vi "Write To FPGA.vi"(7 "Sample Rate":dbl, 8 "error in (no error)":errorcluster, 9 "Changed?":bool[](array[boolean]), 10 "Values":dbl[](array[numeric]), 11 "FPGA Refs":T1 {"Data Type" format="%.0x"}) -> (0 "error out":errorcluster, 2 "Values out":dbl[](array[numeric]), 3 "FPGA Refs":T1 {"Data Type" format="%.0x"})   [LabVIEW 2015, in "Fuel Injection Addon Engine.lvlib"]
uses:
  Fuel Injection Addon Engine.lvlib
  Types/FPGA Refs.ctl
  Shared/Types/FPGA Data Types.ctl
  <vilib>/rvi/errors/niLvFpgaAdjustHostInterfaceError.vi
  <vilib>/Utility/error.llb/Error Cluster From Error Code.vi
  <vilib>/rvi/interface/nirviReadWriteControl/nirviReadWriteControl.xnode
  <vilib>/rvi/interface/Simulation/niFpgaSimulationCallBeginRW.vi
  NiFpgaLv.dll
  Shared/Fuel Injection Addon Shared.lvlib
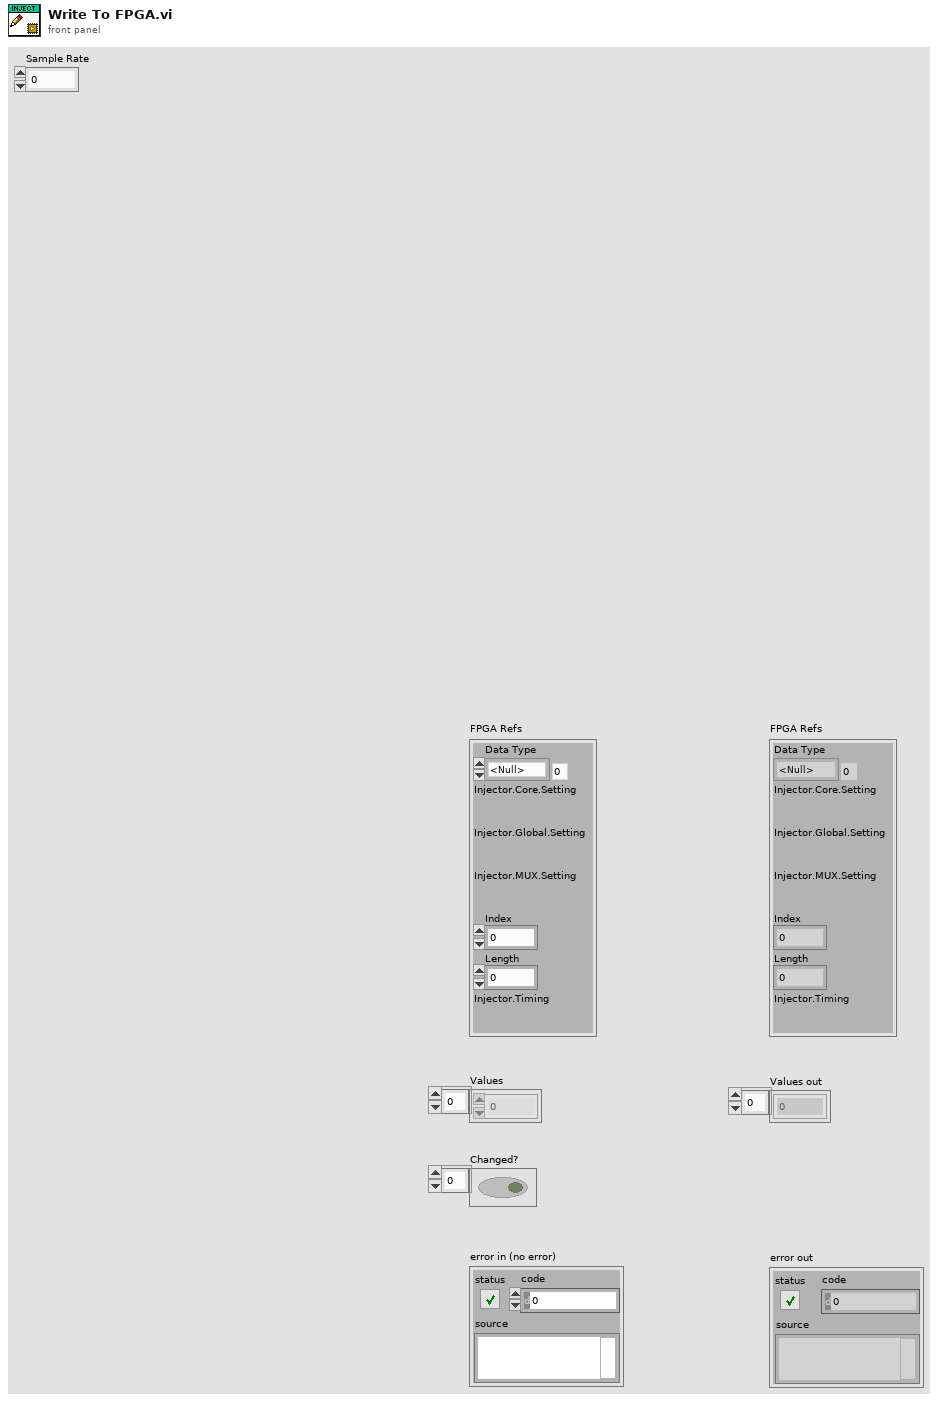
[diagram p1: front panel]
types:
  T1 = typedef "Fuel Injection Addon Engine.lvlib/FPGA Refs.ctl" = cluster{"Data Type":T2, "Injector.Core.Setting":refnum<k20>, "Injector.Global.Setting":refnum<k20>, "Injector.MUX.Setting":refnum<k20>, "Index":i32, "Length":i32, "Injector.Timing":refnum<k20>}
  T2 = typedef "Fuel Injection Addon Shared.lvlib/FPGA Data Types.ctl" = enum8{"<Null>", "Injector.Core.Setting", "Injector.Global.Setting", "Injector.Mux.Setting", "Injector.Timing"}
  T3 = cluster{"Voltage Offset":fxp<+/-,32,8>, "Current Offset":fxp<+/-,32,8>}
  T4 = cluster{"Enable?":bool, "Initial Voltage Threshold":fxp<+/-,32,8>, "Event Dwell Limit":u16, "Voltage Gain":fxp<+/-,32,8>, "Current Gain":fxp<+/-,32,8>, "Filter Samples":u8, "Pretrigger Samples":u8}
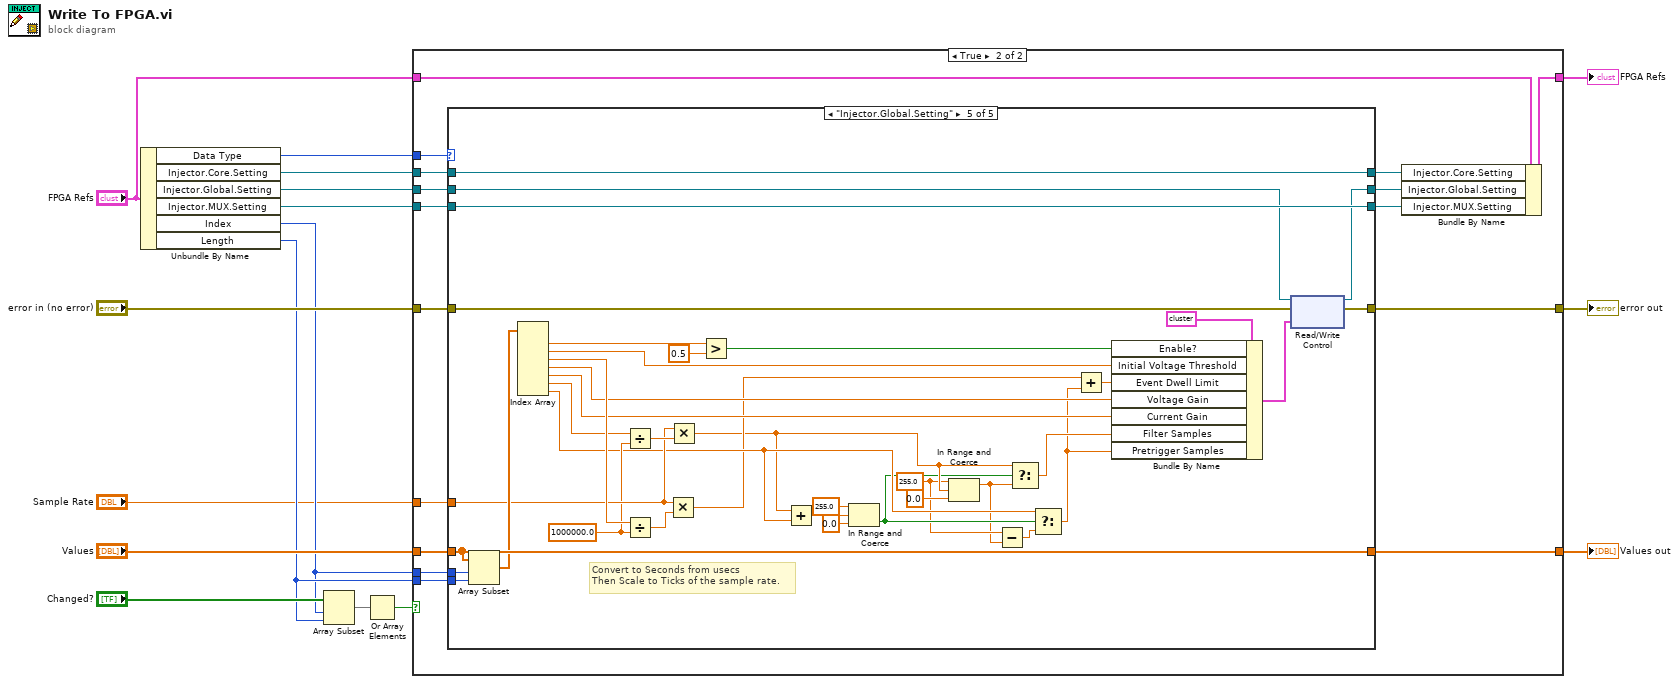
[diagram p0: block diagram]
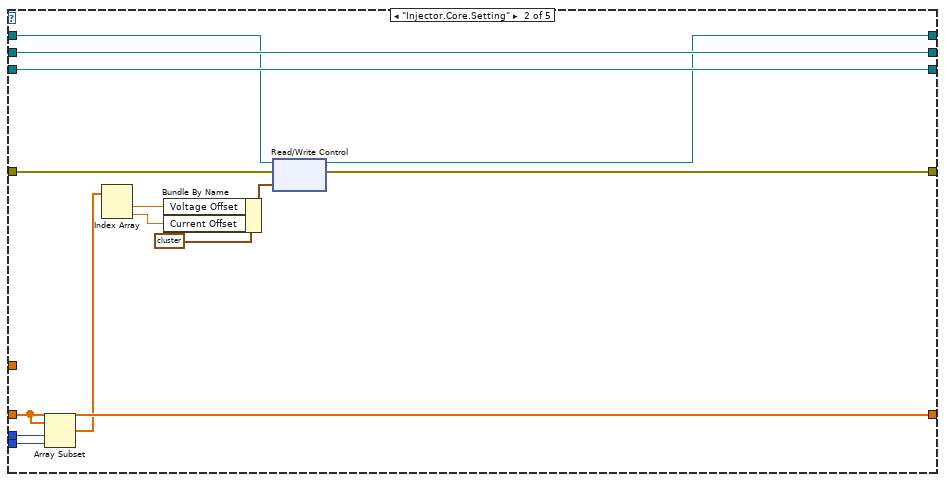
[diagram p4: hidden frame]
diagram:
  n1 = Unbundle By Name("FPGA Refs") -> ("Data Type"=w16:T2, "Injector.Core.Setting"=w7:refnum<k20>, "Injector.Global.Setting"=w11:refnum<k20>, "Injector.MUX.Setting"=w12:refnum<k20>, "Index"=w2:i32, "Length"=w3:i32)
  n2 = Array Subset(array="Changed?", index=w2, length=w3) -> (w9:bool[])
  n3 = Or Array Elements(Boolean array=w9) -> (logical OR=w8:bool)
  n4 = case shown="True" w8 {
    tunnel: w16 -> [_ w35]
    tunnel: "error in (no error)" -> [w18 w34]
    tunnel: [w18 w33] -> w15
    tunnel: "FPGA Refs" -> [w19 w32]
    tunnel: [w19 w31] -> w4
    tunnel: [w17 w30] -> w14
    tunnel: "Values" -> [w17 w29]
    tunnel: w12 -> [_ w28]
    tunnel: w11 -> [_ w25]
    tunnel: w2 -> [_ w24]
    tunnel: w3 -> [_ w23]
    tunnel: w7 -> [_ w22]
    tunnel: "Sample Rate" -> [_ w20]
    frame False {
    }
    frame True {
      n5 = case shown="\"Injector.Global.Setting\"" w35 {
        tunnel: w34 -> [w40 w53 w57 w62 w102]
        tunnel: [w40 w52 w57 w62 w101] -> w33
        tunnel: [w39 w49 w58 w63 w98] -> w30
        tunnel: w29 -> [w39 w49 w58 w63 w98]
        tunnel: w23 -> [_ w50 _ _ w99]
        tunnel: w24 -> [_ w51 _ _ w100]
        tunnel: w28 -> [w38 w47 w55 w60 w96]
        tunnel: [w38 w47 w55 w60 w96] -> w27
        tunnel: [w37 w54 w59 w64 w91] -> w26
        tunnel: w25 -> [w37 w54 w59 w64 w92]
        tunnel: w22 -> [w36 w46 w56 w61 w93]
        tunnel: [w36 w45 w56 w61 w93] -> w21
        tunnel: w20 -> [_ _ _ _ w80]
        frame "<Null>", Default {
        }
        frame "Injector.Core.Setting" {
          n6 = Array Subset(array=w49, index=w51, length=w50) -> (w48:dbl[])
          n7 = Index Array(array=w48) -> (element #1=w42:dbl, element #2=w41:dbl)  [unwired: 2 in]
          n8 = Bundle By Name(cluster=T3 {"Voltage Offset"=0.0, "Current Offset"=0.0} ("Value"), "Voltage Offset"=w42, "Current Offset"=w41) -> (w43:T3)
          n9 = xnode "Read/Write Control"("FPGA VI Reference In"=w46, "error in"=w53, "Value"=w43) -> ("FPGA VI Reference Out"=w45:refnum<k20>, "error out"=w52:errorcluster)
        }
        frame "Injector.Mux.Setting" {
          # "DLE NOTE - Only Set in Init"
        }
        frame "Injector.Timing" {
          # "DLE NOTE - Only Set in Init"
        }
        frame "Injector.Global.Setting" {
          w67 = 255.0 ("upper limit")
          w79 = 1000000.0 ("y")
          # "Convert to Seconds from usecs\nThen Scale to Ticks of the sample rate."
          n10 = Array Subset(array=w98, index=w100, length=w99) -> (w97:dbl[])
          n11 = Index Array(array=w97) -> (element #1=w95:dbl, element #2=w94:dbl, element #3=w87:dbl, element #4=w86:dbl, element #5=w85:dbl, element #6=w81:dbl, element #7=w74:dbl)  [unwired: 7 in]
          n12 = Divide(x=w81, y=w79) -> (x/y=w82:dbl)
          n13 = Divide(x=w87, y=w79) -> (x/y=w88:dbl)
          n14 = Multiply(x=w80, y=w88) -> (x*y=w73:dbl)
          n15 = Multiply(x=w80, y=w82) -> (x*y=w69:dbl)
          n16 = Greater?(x=w95, y=0.5 ("x")) -> (0:w90:bool)
          n17 = Add(x=w69, y=w74) -> (x+y=w78:dbl)
          n18 = In Range and Coerce(upper limit=255.0, x=w78, lower limit=0.0) -> (In Range?=w68:bool)  [unwired: 1 out]
          n19 = In Range and Coerce(upper limit=w67, x=w69, lower limit=0.0) -> (coerced(x)=w66:dbl)  [unwired: 1 out]
          n20 = Subtract(x=w67, y=w66) -> (x-y=w65:dbl)
          n21 = Select(t=w69, s=w68, f=w66) -> (s? t:f=w75:dbl)
          n22 = Select(t=w74, s=w68, f=w65) -> (s? t:f=w71:dbl)
          n23 = Add(x=w73, y=w71) -> (x+y=w72:dbl)
          n24 = Bundle By Name(cluster=T4 {"Enable?"=FALSE, "Initial Voltage Threshold"=0.0, "Event Dwell Limit"=0, "Voltage Gain"=0.0, "Current Gain"=0.0, "Filter Samples"=0, "Pretrigger Samples"=0} ("Value"), "Enable?"=w90, "Initial Voltage Threshold"=w94, "Event Dwell Limit"=w72, "Voltage Gain"=w86, "Current Gain"=w85, "Filter Samples"=w75, "Pretrigger Samples"=w71) -> (w83:T4)
          n25 = xnode "Read/Write Control"("FPGA VI Reference In"=w92, "error in"=w102, "Value"=w83) -> ("FPGA VI Reference Out"=w91:refnum<k20>, "error out"=w101:errorcluster)
        }
      }
      n26 = Bundle By Name(cluster=w32, "Injector.Core.Setting"=w21, "Injector.Global.Setting"=w26, "Injector.MUX.Setting"=w27) -> (w31:T1)
    }
  }
  "FPGA Refs" <- w4
  "error out" <- w15
  "Values out" <- w14
